vi "Get Window Image From HWND.vi"(8 "error in (no error)":errorcluster, 10 "Window Name (\"\")":string, 11 "HWnd":u32) -> (0 "error out":errorcluster, 3 "Window Image":T1)   [LabVIEW 2014]
doc: "This VI will return a print screem image <B>Window Image</B> from the window with the handle <B>HWnd</B> or window title of <B>Window Name (\"\")</B>.\n\nThis will not function properly if the window is hidden or not open."
uses:
  <vilib>/picture/picture.llb/imagedata.ctl
  System.Drawing
  <userlib>/_OpenG.lib/error/error.llb/Build Error Cluster__ogtk.vi
  user32.dll
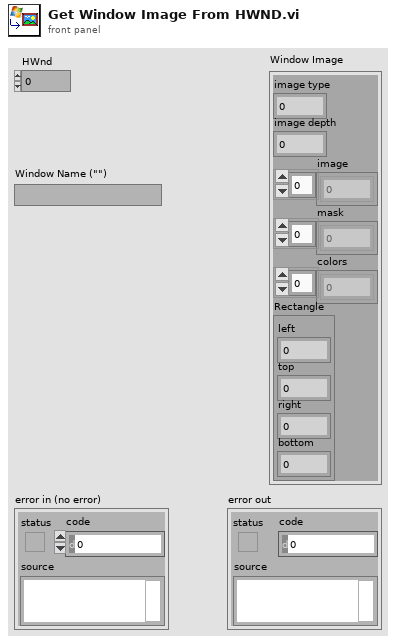
[diagram p1: front panel]
types:
  T1 = typedef "imagedata.ctl" = cluster{"image type":i32, "image depth":i32, "image":u8[], "mask":u8[], "colors":u32[], "Rectangle":cluster{"left":i16, "top":i16, "right":i16, "bottom":i16}}
  T2 = typedef "Window Rectangle (hwnd).ctl" = cluster{"left":i16, "top":i16, "right":i16, "bottom":i16}
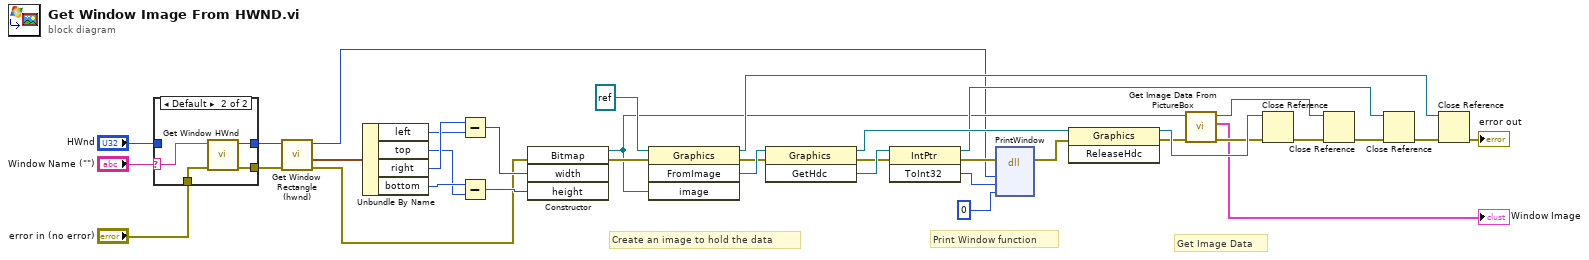
[diagram p0: block diagram]
diagram:
  # "Get Image Data"
  # "Print Window function"
  # "Create an image to hold the data"
  n1 = case shown="Default" "Window Name (\"\")" {
    selector: "Window Name (\"\")" -> [_ w40]
    tunnel: "error in (no error)" -> [w38 w43]
    tunnel: [w39 w42] -> w4
    tunnel: "HWnd" -> [w39 _]
    tunnel: [w38 w41] -> w2
    frame "" {
    }
    frame Default {
      n2 = call "Get Window HWnd.vi"("error in (no error)"=w43, "Window Name"=w40) -> ("error out"=w41:errorcluster, "HWnd Out"=w42:u32)  [unwired: 8 in]
    }
  }
  n3 = call "Get Window Rectangle (hwnd).vi"("error in (no error)"=w2, "HWnd"=w4) -> ("error out"=w9:errorcluster, "Window Rect"=w17:T2, "HWnd Out"=w6:u32)  [unwired: 7 in]
  n4 = Unbundle By Name(w17) -> ("left"=w15:i16, "top"=w13:i16, "right"=w16:i16, "bottom"=w14:i16)
  n5 = Subtract(x=w16, y=w15) -> (x-y=w12:i16)
  n6 = Subtract(x=w14, y=w13) -> (x-y=w11:i16)
  n7 = constructor class="Bitmap"(error in=w9, "width"=w12, "height"=w11) -> (reference out=w19:refnum<k24>, error out=w31:errorcluster)  [unwired: 2 in, 3 out]
  n8 = invoke class="Graphics" method="FromImage"(reference=refnum<k24> refnum, error in=w31, "image"=w19) -> (reference out=w22:refnum<k24>, error out=w32:errorcluster, "FromImage"=w37:refnum<k24>)  [unwired: 1 in, 1 out]
  n9 = invoke class="Graphics" method="GetHdc"(reference=w37, error in=w32) -> (reference out=w29:refnum<k24>, error out=w33:errorcluster, "GetHdc"=w35:refnum<k24>)  [unwired: 1 in]
  n10 = invoke class="IntPtr" method="ToInt32"(reference=w35, error in=w33) -> (reference out=w24:refnum<k24>, error out=w30:errorcluster, "ToInt32"=w34:i32)  [unwired: 1 in]
  n11 = dll-call lib="user32.dll" fn="PrintWindow"(error in=w30, "hwnd"=w6, "hdcBlt"=w34, "nFlags"=u32 0) -> (error out=w28:errorcluster)  [unwired: 6 in, 1 out]
  n12 = invoke class="Graphics" method="ReleaseHdc"(reference=w29, error in=w28) -> (reference out=w27:refnum<k24>, error out=w20:errorcluster)  [unwired: 1 in, 1 out]
  n13 = call "Get Image Data From PictureBox.vi"("error in (no error)"=w20, "Image"=w19) -> ("error out"=w10:errorcluster, "Image Data"=→"Window Image":T1, "Image Out"=w18:refnum<k24>)  [unwired: 7 in]
  n14 = Close Reference(reference=w27, error in (no error)=w10) -> (error out=w26:errorcluster)
  n15 = Close Reference(reference=w18, error in (no error)=w26) -> (error out=w25:errorcluster)
  n16 = Close Reference(reference=w24, error in (no error)=w25) -> (error out=w23:errorcluster)
  n17 = Close Reference(reference=w22, error in (no error)=w23) -> (error out=→"error out":errorcluster)
